vi "UHR-Fleezers Control (host) - 11.9b.vi"() -> ()   [LabVIEW 2014] (continued)
                  }
                }
                n3326 = Write to Binary File(file (use dialog)=w5210, data=w5203, 5:FALSE ("prepend array or string size? (T)"), 9:T24."big-endian, network order" ("byte order (0:big-endian, network order)")) -> ()  [unwired: 1 in, 4 out]
                n3327 = feedback #39(w5176) -> (w5178:dbl[])
                n3328 = Build Array (concatenate)(w5178, w5176) -> (w5177:dbl[])
                n3329 = Select(t=w5176, s=w5142, f=w5177) -> (s? t:f=w5162:dbl[])
                n3330 = feedback-in #39(w5162) -> ()
                n3331 = feedback #40(w5184) -> (w5197:dbl[])
                n3332 = Build Array (concatenate)(w5197, w5184) -> (w5196:dbl[])
                n3333 = Select(t=w5184, s=w5142, f=w5196) -> (s? t:f=w5171:dbl[])
                n3334 = feedback-in #40(w5171) -> ()
                n3335 = Divide(x=w5211, y=w5212) -> (x/y=w5214:dbl)
                n3336 = Multiply(x=w5214, y=100.0) -> (x*y=w5213:dbl)
                n3337 = Build Array(w5171, w5162) -> (→"Saved APD":dbl[][])
                n3338 = Array Size(array=w5171) -> (size(s)=w5189:i32)
                n3339 = Unbundle By Name(w5191) -> ("Y"=w5195:dbl[])
                n3340 = Subtract(x=w5189, y="N pts to average") -> (x-y=w5165:i32)
                n3341 = Multiply(x="N pts to average", y=u16 2) -> (x*y=w5166:u16)
                n3342 = Subtract(x=w5189, y=w5166) -> (x-y=w5164:i32)
                n3343 = feedback #41(w5195) -> (w5194:dbl[])
                n3344 = Build Array (concatenate)(w5194, w5195) -> (w5193:dbl[])
                n3345 = Select(t=w5195, s=w5142, f=w5193) -> (s? t:f=w5192:dbl[])
                "Trap Delta Graph" <- w5192
                n3346 = feedback-in #41(w5192) -> ()
                n3347 = Array Subset(array=w5171, index=w5165, length="N pts to average") -> (w5188:dbl[])
                n3348 = Array Subset(array=w5171, index=w5164, length="N pts to average") -> (w5187:dbl[])
                n3349 = Array Subset(array=w5162, index=w5165, length="N pts to average") -> (w5168:dbl[])
                n3350 = Array Subset(array=w5162, index=w5164, length="N pts to average") -> (w5167:dbl[])
                n3351 = Index Array(array=w5145, index=0) -> (element=w5143:waveform(dbl))
                n3352 = call-poly <vilib>:"Mean.vi"("X"=w5188) -> ("mean"=w5186:dbl)  [unwired: 1 out]
                n3353 = call-poly <vilib>:"Mean.vi"("X"=w5168) -> ("mean"=w5161:dbl)  [unwired: 1 out]
                n3354 = call-poly <vilib>:"Mean.vi"("X"=w5187) -> ("mean"=w5185:dbl)  [unwired: 1 out]
                n3355 = call-poly <vilib>:"Mean.vi"("X"=w5167) -> ("mean"=w5160:dbl)  [unwired: 1 out]
                n3356 = Unbundle By Name(w5143) -> ("Y"=w5140:dbl[])
                n3357 = Subtract(x=w5161, y=w5160) -> (x-y=w5152:dbl)
                "Delta Fl. 2" <- w5152
                n3358 = Subtract(x=w5186, y=w5185) -> (x-y=w5183:dbl)
                "Delta Fl. 1" <- w5183
                n3359 = Initialize Array(w5183, 1 ("dimension size")) -> (w5180:dbl[])
                n3360 = Initialize Array(w5152, 1 ("dimension size")) -> (w5157:dbl[])
                n3361 = feedback #42(w5180) -> (w5181:dbl[])
                n3362 = Build Array (concatenate)(w5181, w5180) -> (w5179:dbl[])
                n3363 = feedback #43(w5157) -> (w5158:dbl[])
                n3364 = Build Array (concatenate)(w5158, w5157) -> (w5156:dbl[])
                n3365 = feedback #44(w5140) -> (w5139:dbl[])
                n3366 = Build Array (concatenate)(w5139, w5140) -> (w5141:dbl[])
                n3367 = Select(t=w5140, s=w5142, f=w5141) -> (s? t:f=w5138:dbl[])
                "Saved trap pos" <- w5138
                n3368 = feedback-in #44(w5138) -> ()
                n3369 = Select(t=w5180, s=w5142, f=w5179) -> (s? t:f=w5155:dbl[])
                n3370 = feedback-in #42(w5155) -> ()
                n3371 = Select(t=w5157, s=w5142, f=w5156) -> (s? t:f=w5154:dbl[])
                n3372 = feedback-in #43(w5154) -> ()
                n3373 = Build Array(w5155, w5154) -> (→"Save APD Deriv":dbl[][])
              }
            }
            "Progress" <- w5121
            "Progress 2" <- w5121
          }
        }
      }
    }
    n3374 = Bundle By Name(cluster=w3716, "Green FB Ch 0"=w3715, "Green FB Ch 1"=w3714) -> (w3694:T48)
    "Green FB Signals (V)" <- w3694
    n3375 = Unbundle By Name(w3694) -> ("Green FB Ch 2"=→"Green FB Plot":dbl)
    n3376 = local read "wait to reset values"() -> (w3783:bool)
    n3377 = Not(x=w3781) -> (.not. x?=w3784:bool)
    n3378 = And(x=w3784, y=w3783) -> (x .and. y?=w3785:bool)
    n3379 = case "Part of MCL raster scanning: returns to initial positions after scan done" shown="True" w3785 {
      tunnel: w3503 -> [w4656 w4663]
      tunnel: [w4656 w4662] -> w3787
      tunnel: w3502 -> [w4655 w4661]
      tunnel: [w4655 w4660] -> w3782
      frame False {
      }
      frame True {
        w4671 = 10.0 ("y")
        w4670 = 32767.0 ("y")
        # "to return scan values\nafter a synchronous \nAOM scan"
        n3380 = local read "AO2"() -> (w4664:dbl)
        n3381 = local read "AO1"() -> (w4665:dbl)
        n3382 = local write "wait to reset values"(FALSE ("wait to reset values")) -> ()
        n3383 = Multiply(x=w4665, y=w4670) -> (x*y=w4667:dbl)
        n3384 = Multiply(x=w4664, y=w4670) -> (x*y=w4669:dbl)
        n3385 = Divide(x=w4667, y=w4671) -> (x/y=w4666:dbl)
        n3386 = Divide(x=w4669, y=w4671) -> (x/y=w4668:dbl)
        n3387 = To Word Integer(number=w4666) -> (16bit integer=w4672:i16)
        n3388 = To Word Integer(number=w4668) -> (16bit integer=w4673:i16)
        n3389 = local read "Total Counts (ticks)"() -> (w4657:u32)
        n3390 = xnode "Read/Write Control"("FPGA VI Reference In"=w4663, "error in"=w4661, "AO1"=w4672, "AO2"=w4673, "MCL count"=w4657) -> ("FPGA VI Reference Out"=w4662:T19, "error out"=w4660:errorcluster)
        n3391 = local read "Scan Range (V)\n(of steps)"() -> (w4658:dbl)
        n3392 = property on="Scan Range (V)\n(of steps)" class="DigNum (strict)"("Val(Sgnl)"=w4658) -> ()  [unwired: 2 in, 2 out]
      }
    }
    n3393 = node-c288() -> ()  [unwired: 2 out]
  }
  n3394 = VISA Close(VISA resource name=w104, error in (no error)=w103) -> (error out=w151:errorcluster)
  n3395 = call <vilib>:"Simple Error Handler.vi"("error in (no error)"=w151) -> ()  [unwired: 1 in, 8 out]
  n3396 = node-c288(w110) -> ()  [unwired: 1 out]
  n3397 = node-c288(w195) -> ()  [unwired: 1 out]
  n3398 = flat-sequence {
    tunnel: w287 -> [w5258]
    tunnel: w289 -> [w5259]
    tunnel: [w5257] -> w268
    tunnel: [w5256] -> w267
    tunnel: w251 -> [_]
    tunnel: w203 -> [_]
    tunnel: w116 -> [_]
    tunnel: w268 -> [w5260]
    tunnel: w267 -> [w5261]
    frame #0 {
      w5255 = FALSE ("AI to FIFO")
      n3399 = xnode "Read/Write Control"("FPGA VI Reference In"=w5259, "error in"=w5258, "AI to FIFO"=w5255, "APD to FIFO"=w5255) -> ("FPGA VI Reference Out"=w5257:T19, "error out"=w5256:errorcluster)
    }
    frame #1 {
      n3400 = xnode "Close FPGA VI Reference"("FPGA VI Reference In"=w5260, "error in"=w5261) -> ("error out"=→"error out":errorcluster)
    }
  }
